vi "FTW-SQLite-Core-PrepareStatement.vi"(0 "SQLite Connection":refnum<data-value>, 5 "SQL Statement":string, 11 "error in":errorcluster) -> (2 "Begin Timestamp":dbl format="%.3fmsec\n%<%D:%H:%M:%S%3u>t", 3 "Compile Time":dbl format="%.4psec", 4 "SQLite Connection out":refnum<data-value>, 6 "SQLite Library Filepath":path, 8 "Prepared Statements":i64[](array[numeric]) format="0x%016x", 15 "error out":errorcluster)   [LabVIEW 2014]
uses:
  FTW-SQLite-Core-Structure.ctl
  error/FTW-ERR-ThrowGenericError.vi
  error/FTW-ERR-ThrowError.vi
  error/FTW-ERR-NoErrorConstant.vi
  string/FTW-STR-ReplaceWhitespace.vi
  error/FTW-ERR-CallChain.vi
panel:
  # "Inputs"
  # "Outputs"
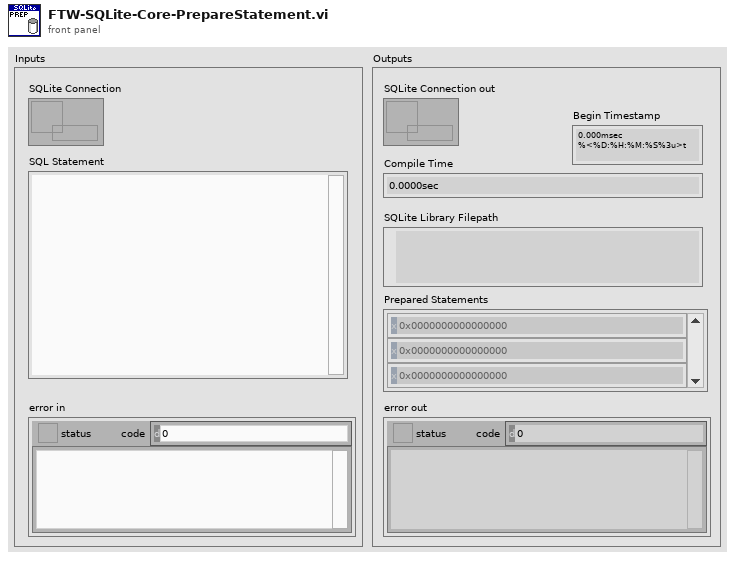
[diagram p1: front panel]
types:
  T1 = typedef "FTW-SQLite-Core-Structure.ctl" = cluster{"Connection":u64}
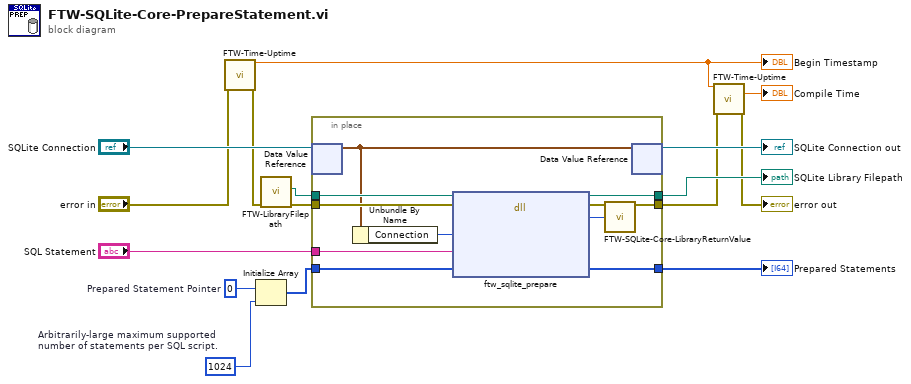
[diagram p0: block diagram]
diagram:
  w3 = 1024  # Arbitrarily-large maximum supported number of statements per SQL script.
  w2 = i64 0  # Prepared Statement Pointer
  n1 = call "FTW-Time-Uptime.vi"("error in"="error in") -> ("Current Uptime"=w6:dbl, "error out"=w10:errorcluster)  [unwired: 12 in, 1 out]
  "Begin Timestamp" <- w6
  n2 = Initialize Array(w2, w3) -> (w1:i64[])
  n3 = call "FTW-LibraryFilepath.vi"("error in"=w10) -> ("error out"=w4:errorcluster, "Library Filepath"=w5:path)  [unwired: 8 in, 1 out]
  n4 = in-place {
    in-place-border: [w27] -> w9
    in-place-border: "SQL Statement" -> [w26]
    in-place-border: w5 -> [w24]
    in-place-border: w4 -> [w23]
    in-place-border: [w19] -> w14
    in-place-border: [w18] -> w13
    in-place-border: w1 -> [w17]
    n5 = in-place-dvr #1("SQLite Connection") -> (w22:T1)  [unwired: 1 out]
    n6 = Unbundle By Name(w22) -> ("Connection"=w25:u64)
    n7 = dll-call lib="?" fn="ftw_sqlite_prepare"(path in=w24, error in=w23, "Connection Handle"=w25, "SQL Script"=w26, "Statements"=w17) -> (path out=w18:path, error out=w21:errorcluster, "Return Value"=w20:i32, "Statements"=w19:i64[])  [unwired: 3 in]
    n8 = call "FTW-SQLite-Core-LibraryReturnValue.vi"("error in"=w21, "Return Value"=w20) -> ("error out"=w27:errorcluster)  [unwired: 13 in]
    n9 = in-place-dvr #1(w22) -> (→"SQLite Connection out":refnum<data-value>)  [unwired: 1 out]
  }
  "Prepared Statements" <- w14
  "SQLite Library Filepath" <- w13
  n10 = call "FTW-Time-Uptime.vi"("Previous Uptime"=w6, "error in"=w9) -> ("Elapsed Time"=→"Compile Time":dbl, "error out"=→"error out":errorcluster)  [unwired: 11 in, 1 out]
